vi "SetUpMotor.vi"(8 "Error In":errorcluster, 10 "Serial Number":string="27004535", 11 "LabJack in":refnum<k24>) -> (0 "Error Out":errorcluster, 3 "LabJack out":refnum<k24>)   [LabVIEW 2018, in "ThorlabsLabJack.lvlib" / "ThorlabsLabJack.lvclass"]
uses:
  ThorlabsLabJack.lvclass
  C:/Projects/LabVIEW/In-Progress/Chetan Malpure/Axis/Thorlabs LabJack/Drivers/Thorlabs.MotionControl.IntegratedStepperMotorsCLI.dll
  Drivers/Thorlabs.MotionControl.IntegratedStepperMotorsCLI.dll
  C:/Projects/LabVIEW/In-Progress/Chetan Malpure/Axis/Thorlabs LabJack/Drivers/Thorlabs.MotionControl.GenericMotorCLI.dll
  Drivers/Thorlabs.MotionControl.GenericMotorCLI.dll
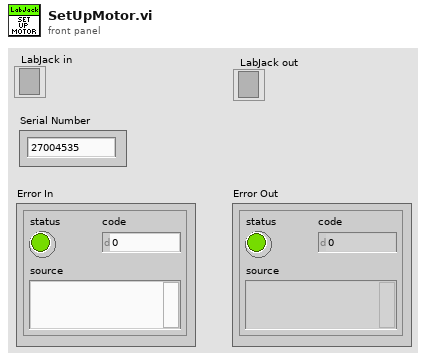
[diagram p1: front panel]
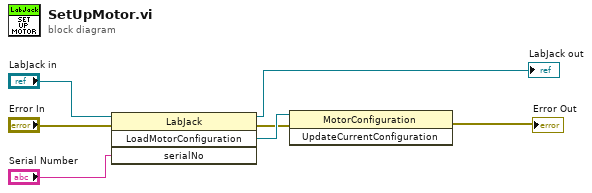
[diagram p0: block diagram]
diagram:
  n1 = invoke class="LabJack" method="LoadMotorConfiguration"(reference="LabJack in", error in="Error In", "serialNo"="Serial Number") -> (reference out=→"LabJack out":refnum<k24>, error out=w4:errorcluster, "LoadMotorConfiguration"=w5:refnum<k24>)  [unwired: 1 in, 1 out]
  n2 = invoke class="MotorConfiguration" method="UpdateCurrentConfiguration"(reference=w5, error in=w4) -> (error out=→"Error Out":errorcluster)  [unwired: 1 in, 2 out]
